vi "Add_Core.vi"(6 "Options":T1={"DbType"=-1, "Direction"=-1, "Size"=-1, "Precision"=255, "Scale"=255} {"Direction" items=["Input"=1, "Output"=2, "InputOutput"=3, "ReturnValue"=6]; "DbType" items=["AnsiString"=0, "Binary"=1, "Byte"=2, "Boolean"=3, "Currency"=4, "Date"=5, "DateTime"=6, "Decimal"=7, "Double"=8, "Guid"=9, "Int16"=10, "Int32"=11, "Int64"=12, "Object"=13, "SByte"=14, "Single"=15, "String"=16, "Time"=17, "UInt16"=18, "UInt32"=19, "UInt64"=20, "VarNumeric"=21, "AnsiStringFixedLength"=22, "StringFixedLength"=23, "Xml"=25, "DateTime2"=26, "DateTimeOffset"=27]}, 8 "error in (no error)":errorcluster, 9 "value":variant, 10 "name":string, 11 "DynamicParameters in":refnum<class "DynamicParameters.lvclass">) -> (0 "error out":errorcluster, 3 "DynamicParameters out":refnum<class "DynamicParameters.lvclass">)   [LabVIEW 2020, in "ORM.lvlib" / "DynamicParameters.lvclass"]
uses:
  DynamicParameters.lvclass
  DynamicParameters.lvclass/DynamicParameters.ctl
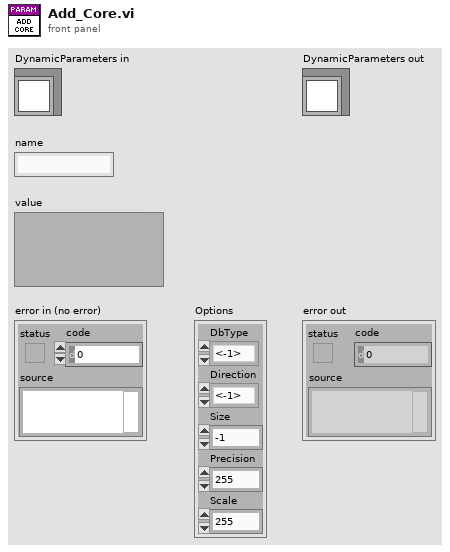
[diagram p1: front panel]
types:
  T1 = cluster{"DbType":i32, "Direction":i32, "Size":i32, "Precision":u8, "Scale":u8}
  T2 = cluster{"DbType":i32, "Direction":i32, "Size":i32, "Precision":u8, "Scale":u8}[]
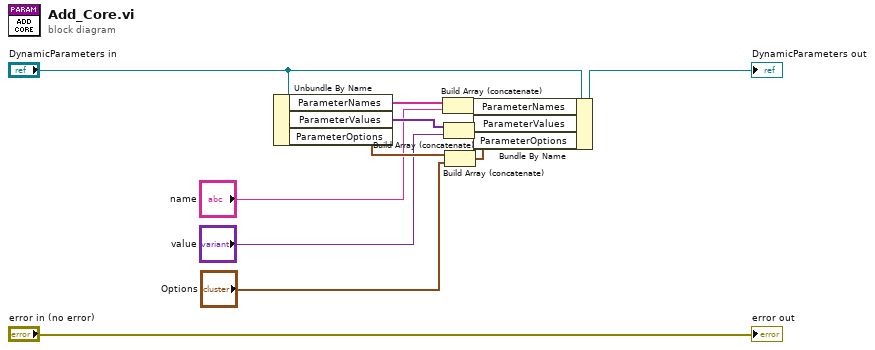
[diagram p0: block diagram]
diagram:
  n1 = Unbundle By Name("DynamicParameters in") -> ("ParameterNames"=w11:string[], "ParameterValues"=w10:variant[], "ParameterOptions"=w9:T2)
  n2 = Build Array (concatenate)(w11, "name") -> (w5:string[])
  n3 = Build Array (concatenate)(w10, "value") -> (w4:variant[])
  n4 = Build Array (concatenate)(w9, "Options") -> (w3:T2)
  n5 = Bundle By Name(cluster="DynamicParameters in", "ParameterNames"=w5, "ParameterValues"=w4, "ParameterOptions"=w3) -> (→"DynamicParameters out":refnum<class "DynamicParameters.lvclass">)
  "error out" <- "error in (no error)"
